vi "Main.vi"() -> ()   [LabVIEW 2019]
uses:
  Asset Location/Asset Location.lvclass
  Asset External Calibration/Asset External Calibration.lvclass
  Asset/Asset.lvclass
panel:
  in  "Calibration Comments":string
  in  "Recommended Calibration Interval":u32
  in  "Calibration Date (UTC)":timestamp format="%<%H:%M:%S%3u\n%Y/%m/%d>T"
  in  "Supports Calibration":bool
  in  "Parent":string
  in  "Slot Number":u32
  in  "Hardware Version":string
  in  "Firmware Version":string
  in  "Model Number":u32
  in  "Model Name":string
  in  "Vendor Number":u32
  in  "Vendor Name":string
  in  "Serial Number":string
  in  "Asset Name":string
  in  "Bus Type":T1(ring)
  in  "Asset Class":enum16{"Undefined", "Asset", "Dut", "Fixture"}(ring)
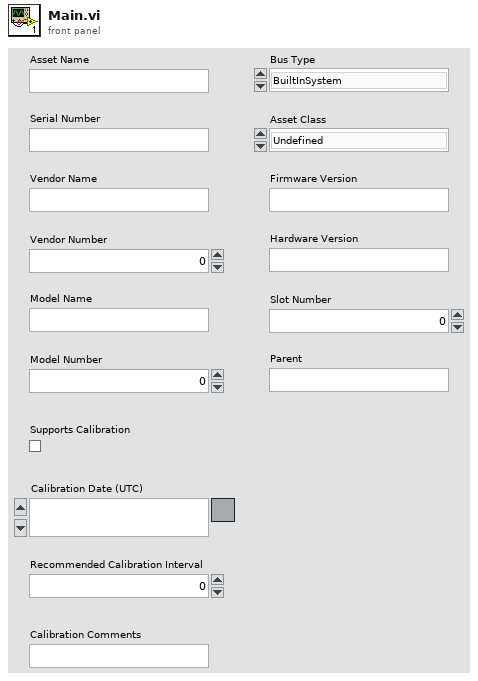
[diagram p1: front panel]
types:
  T1 = enum16{"BuiltInSystem", "PciPxi", "Usb", "Gpib", "Vxi", "Serial", "TcpIp", "cRio", "Scxi", "cDaq", "SwitchBlock", "Scc", "FireWire", "Accessory", "Can", "SwitchBlockDevice"}
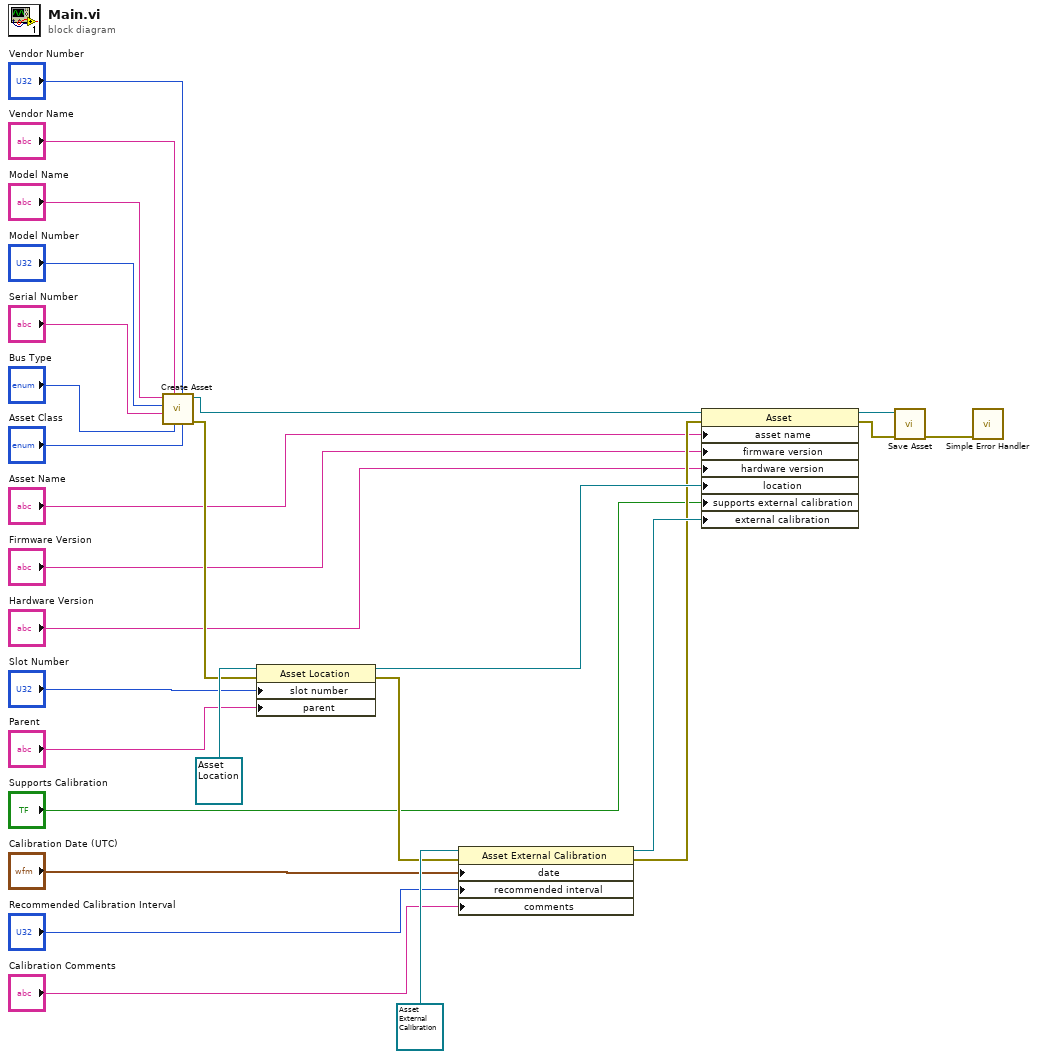
[diagram p0: block diagram]
diagram:
  n1 = call "Create Asset.vi"("Asset Class"="Asset Class", "Vendor Number"="Vendor Number", "Bus Type"="Bus Type", "Vendor Name"="Vendor Name", "Serial Number"="Serial Number", "Model Number"="Model Number", "Model Name"="Model Name") -> ("Error Out"=w18:errorcluster, "Asset"=w25:refnum<class "Asset.lvclass">)  [unwired: 3 in]
  n2 = property class="Asset Location"(reference=refnum<class "Asset Location.lvclass"> refnum ("AssetLocation.lvclass"), error in=w18, "slot number"="Slot Number", "parent"="Parent") -> (reference out=w22:refnum<class "Asset Location.lvclass">, error out=w17:errorcluster)
  n3 = property class="Asset External Calibration"(reference=refnum<class "Asset External Calibration.lvclass"> refnum ("AssetExternalCalibration.lvclass"), error in=w17, "date"="Calibration Date (UTC)", "recommended interval"="Recommended Calibration Interval", "comments"="Calibration Comments") -> (reference out=w21:refnum<class "Asset External Calibration.lvclass">, error out=w16:errorcluster)
  n4 = property class="Asset"(reference=w25, error in=w16, "asset name"="Asset Name", "firmware version"="Firmware Version", "hardware version"="Hardware Version", "location"=w22, "supports external calibration"="Supports Calibration", "external calibration"=w21) -> (reference out=w20:refnum<class "Asset.lvclass">, error out=w19:errorcluster)
  n5 = call "Save Asset.vi"("Error In"=w19, "Asset"=w20) -> ("Error Out"=w1:errorcluster)  [unwired: 9 in]
  n6 = call <vilib>:"Simple Error Handler.vi"("error in (no error)"=w1) -> ()  [unwired: 4 in, 5 out]
